vi "SHAPE_decodeParameters.vi"(3 "Parameters":i32[](array[numeric]), 5 "BandGlobalOpt.lvclass":refnum<class "Shapelets Search GA.lvclass">) -> (0 "Shapelet":dbl[][](array[numeric]), 2 "Accuracy":sgl format="%.2f")   [LabVIEW 2016, in "Shapelets Search (GA).lvlib" / "Shapelets Search GA.lvclass"]
uses:
  Shapelets Search GA.lvclass
  Shapelets Search GA.lvclass/Shapelets Search GA.ctl
  <vilib>/Analysis/baseanly.llb/Normalize Vector.vi
  _Shapelets Search (Brute Force)/Shapelets Search (Brute Force).lvlib
  <vilib>/Analysis/NI_AALBase.lvlib
panel:
  # "This VI is a part of BCI Design library, http://www.ru-bci.org \nCopyright © 2020, Sotnikov Peter, All rights reserved. License: GNU GPLv3"
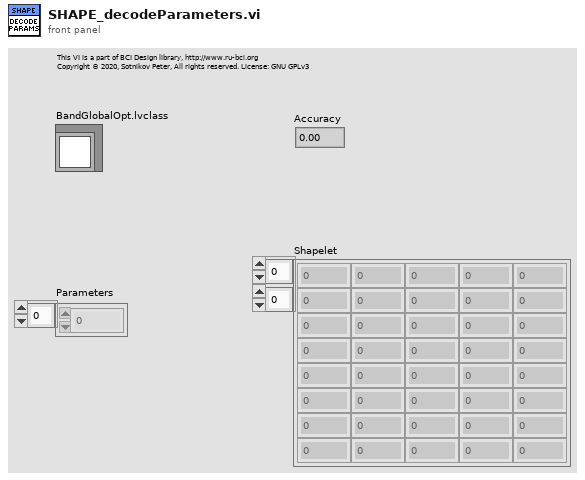
[diagram p1: front panel]
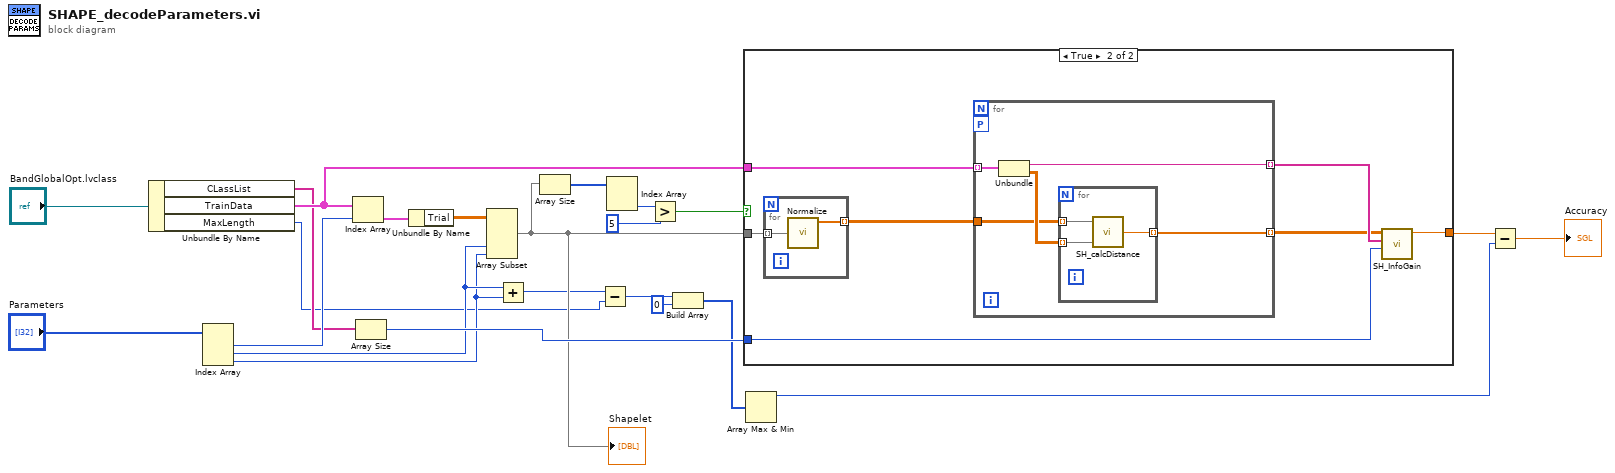
[diagram p0: block diagram]
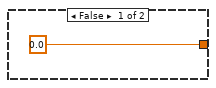
[diagram p2: hidden frame]
diagram:
  n1 = Unbundle By Name("BandGlobalOpt.lvclass") -> ("CLassList"=w18:string[], "TrainData"=w19:cluster{"ClassLabel":string, "Trial":dbl[][]}[], "MaxLength"=w7:i32)
  n2 = Index Array(array="Parameters") -> (element #1=w22:i32, element #2=w11:i32, element #3=w10:i32)  [unwired: 3 in]
  n3 = Index Array(array=w19, index=w22) -> (element=w21:cluster{"ClassLabel":string, "Trial":dbl[][]})
  n4 = Array Size(array=w18) -> (size(s)=w17:i32)
  n5 = Unbundle By Name(w21) -> ("Trial"=w20:dbl[][])
  n6 = Array Subset(array=w20, index (col)=w11, length (col)=w10) -> (w16:dbl[][])  [unwired: 2 in]
  "Shapelet" <- w16
  n7 = Add(x=w11, y=w10) -> (x+y=w8:i32)
  n8 = Array Size(array=w16) -> (size(s)=w15:i32[])
  n9 = Subtract(x=w8, y=w7) -> (x-y=w6:i32)
  n10 = Index Array(array=w15) -> (element #2=w13:i32)  [unwired: 2 in, 1 out]
  n11 = Greater?(x=w13, y=5) -> (0:w9:bool)
  n12 = Build Array(w6, 0 ("element")) -> (w4:i32[])
  n13 = case shown="True" w9 {
    tunnel: w19 -> [_ w30]
    tunnel: w17 -> [_ w28]
    tunnel: w16 -> [_ w27]
    tunnel: [sgl 0.0 ("Accuracy") w26] -> w2
    frame False {
    }
    frame True {
      n14 = for {
        tunnel: [w41] -> w31 mode=indexing
        tunnel: w27 -> [w40] mode=indexing
        n15 = call-poly <vilib>:"Normalize.vi"("Vector"=w40) -> ("Normalized Vector"=w41:dbl[])  [unwired: 1 in, 3 out]
      }
      n16 = for {
        tunnel: w30 -> [w36] mode=indexing
        tunnel: w31 -> [w34]
        workers-P: _ -> [_]
        tunnel: [w33] -> w29 mode=indexing
        tunnel: [w32] -> w25 mode=indexing
        n17 = Unbundle(w36) -> ("ClassLabel"=w33:string, "Trial"=w35:dbl[][])
        n18 = for {
          tunnel: w35 -> [w38] mode=indexing
          tunnel: w34 -> [w39] mode=indexing
          tunnel: [w37] -> w32 mode=indexing
          n19 = call "SH_calcDistance.vi"("Time series"=w38, "Shapelet (normalized)"=w39) -> ("Distance out"=w37:dbl)  [unwired: 1 in]
        }
      }
      n20 = call "SH_InfoGain.vi"("NumberOfClasses"=w28, "Class Labels"=w29, "Distancies"=w25) -> ("Accuracy"=w26:sgl)  [unwired: 7 in, 1 out]
    }
  }
  n21 = Array Max & Min(array=w4) -> (max value=w3:i32)  [unwired: 3 out]
  n22 = Subtract(x=w2, y=w3) -> (x-y=→"Accuracy":sgl)
